vi "RelaySwitching.vi"() -> ()   [LabVIEW 2023]
uses:
  <vilib>/Instr/_visa.llb/VISA Configure Serial Port (Instr).vi
panel:
  in  "Boolean 3":bool
  in  "VISA resource name 2":refnum<visa-resource-name>
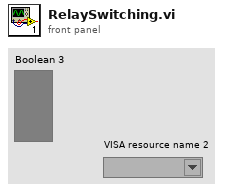
[diagram p1: front panel]
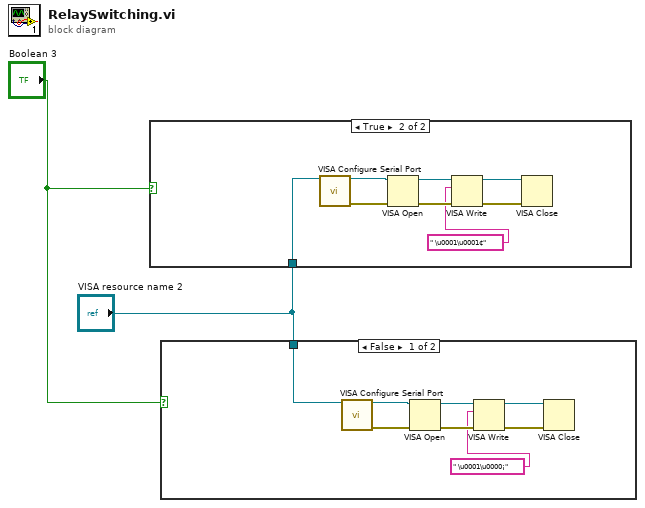
[diagram p0: block diagram]
diagram:
  n1 = case shown="True" "Boolean 3" {
    tunnel: "VISA resource name 2" -> [_ w3]
    frame False {
    }
    frame True {
      n2 = call-poly "VISA Configure Serial Port"("VISA resource name"=w3) -> ("VISA resource name out"=w10:refnum<visa-resource-name>, "error out"=w9:errorcluster)  [unwired: 13 in]
      n3 = VISA Open(error in (no error)=w9, VISA resource name=w10) -> (VISA resource name=w8:refnum<visa-resource-name>, error out=w7:errorcluster)  [unwired: 3 in]
      n4 = VISA Write(VISA resource name=w8, write buffer=" \u0001\u0001¢", error in (no error)=w7) -> (VISA resource name out=w6:refnum<visa-resource-name>, error out=w5:errorcluster)  [unwired: 1 out]
      n5 = VISA Close(VISA resource name=w6, error in (no error)=w5) -> ()  [unwired: 1 out]
    }
  }
  n6 = case shown="False" "Boolean 3" {
    tunnel: "VISA resource name 2" -> [w11 _]
    frame False {
      n7 = call-poly "VISA Configure Serial Port"("VISA resource name"=w11) -> ("VISA resource name out"=w18:refnum<visa-resource-name>, "error out"=w17:errorcluster)  [unwired: 13 in]
      n8 = VISA Open(error in (no error)=w17, VISA resource name=w18) -> (VISA resource name=w16:refnum<visa-resource-name>, error out=w15:errorcluster)  [unwired: 3 in]
      n9 = VISA Write(VISA resource name=w16, write buffer=" \u0001\u0000¡", error in (no error)=w15) -> (VISA resource name out=w14:refnum<visa-resource-name>, error out=w13:errorcluster)  [unwired: 1 out]
      n10 = VISA Close(VISA resource name=w14, error in (no error)=w13) -> ()  [unwired: 1 out]
    }
    frame True {
    }
  }
